vi "InsertData.vi"(4 "Mag B":dbl, 6 "Temp T":dbl, 7 "Time Stamp":timestamp, 8 "error in (no error)":errorcluster, 10 "VNACluster In":T1={"Value"=0.0, "GUI Data Cluster"={"S11"=FALSE, "S21"=FALSE, "S12"=FALSE, "S22"=FALSE, "S11Meas"=enum."Log-magnitude (dB)", "S21Meas"=enum."Log-magnitude (dB)", "S12Meas"=enum."Log-magnitude (dB)", "S22Meas"=enum."Log-magnitude (dB)"}, "Timing"={"Last Operation"=0.0, "Stop @ T"=FALSE, "Delta T Log"=FALSE, "End T"=0.0, "Delta T"=0.0, "Last Temp"=0.0}, "Measurements"=[], "Hardware"={"VNA TCP Con"=refnum, "VNA TCP Port"=5025, "Global T VAR"="", "Global B VAR"=""}, "Operation"={"Operation Mode"=enum."Logging", "Log Folder"=path "", "Measure Mode"=enum."Deltat"}}) -> (0 "error out":errorcluster, 2 "VNACluster Out":T1={"Value"=0.0, "GUI Data Cluster"={"S11"=FALSE, "S21"=FALSE, "S12"=FALSE, "S22"=FALSE, "S11Meas"=enum."Log-magnitude (dB)", "S21Meas"=enum."Log-magnitude (dB)", "S12Meas"=enum."Log-magnitude (dB)", "S22Meas"=enum."Log-magnitude (dB)"}, "Timing"={"Last Operation"=0.0, "Stop @ T"=FALSE, "Delta T Log"=FALSE, "End T"=0.0, "Delta T"=0.0, "Last Temp"=0.0}, "Measurements"=[], "Hardware"={"VNA TCP Con"=refnum, "VNA TCP Port"=5025, "Global T VAR"="", "Global B VAR"=""}, "Operation"={"Operation Mode"=enum."Logging", "Log Folder"=path "", "Measure Mode"=enum."Deltat"}})   [LabVIEW 2021]
uses:
  Sources/Data_Cluster.ctl
  Sources/Measurement_Cluster.ctl
  Sources/Mode_Enum.ctl
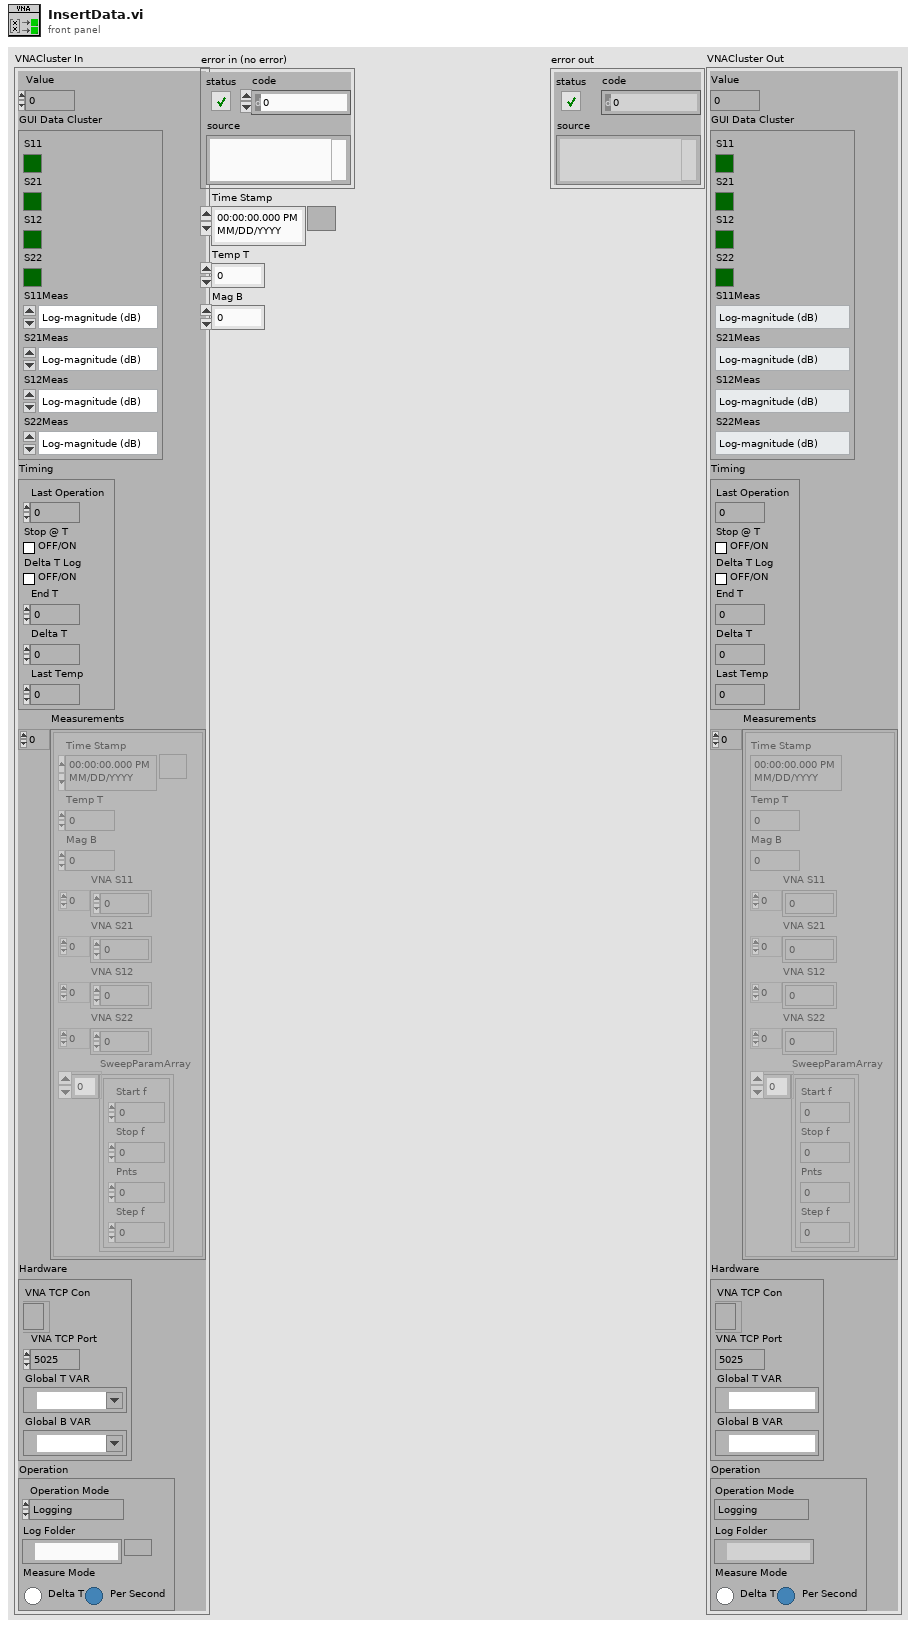
[diagram p1: front panel]
types:
  T1 = typedef "Data_Cluster.ctl" = cluster{"Value":dbl, "GUI Data Cluster":cluster{"S11":bool, "S21":bool, "S12":bool, "S22":bool, "S11Meas":enum16{"Log-magnitude (dB)", "Linear magnitude", "Phase (deg)", "Time Domain", "Real", "Imaginary", "Group Delay", "Polarlinear"}, "S21Meas":enum16{"Log-magnitude (dB)", "Linear magnitude", "Phase (deg)", "Time Domain", "Real", "Imaginary", "Group Delay", "Polarlinear"}, "S12Meas":enum16{"Log-magnitude (dB)", "Linear magnitude", "Phase (deg)", "Time Domain", "Real", "Imaginary", "Group Delay", "Polarlinear"}, "S22Meas":enum16{"Log-magnitude (dB)", "Linear magnitude", "Phase (deg)", "Time Domain", "Real", "Imaginary", "Group Delay", "Polarlinear"}}, "Timing":cluster{"Last Operation":dbl, "Stop @ T":bool, "Delta T Log":bool, "End T":dbl, "Delta T":dbl, "Last Temp":dbl}, "Measurements":T2[], "Hardware":cluster{"VNA TCP Con":refnum<k5>, "VNA TCP Port":i32, "Global T VAR":refnum<k21>, "Global B VAR":refnum<k21>}, "Operation":cluster{"Operation Mode":T3, "Log Folder":path, "Measure Mode":enum32{"DeltaT", "Deltat"}}}
  T2 = typedef "Measurement_Cluster.ctl" = cluster{"Time Stamp":timestamp, "Temp T":dbl, "Mag B":dbl, "VNA S11":dbl[], "VNA S21":dbl[], "VNA S12":dbl[], "VNA S22":dbl[], "SweepParamArray":cluster{"Start f":dbl, "Stop f":dbl, "Pnts":i32, "Step f":dbl}[]}
  T3 = typedef "Mode_Enum.ctl" = enum16{"Logging", "Idle-Off", "Idle"}
  T4 = cluster{"S11":bool, "S21":bool, "S12":bool, "S22":bool, "S11Meas":enum16{"Log-magnitude (dB)", "Linear magnitude", "Phase (deg)", "Time Domain", "Real", "Imaginary", "Group Delay", "Polarlinear"}, "S21Meas":enum16{"Log-magnitude (dB)", "Linear magnitude", "Phase (deg)", "Time Domain", "Real", "Imaginary", "Group Delay", "Polarlinear"}, "S12Meas":enum16{"Log-magnitude (dB)", "Linear magnitude", "Phase (deg)", "Time Domain", "Real", "Imaginary", "Group Delay", "Polarlinear"}, "S22Meas":enum16{"Log-magnitude (dB)", "Linear magnitude", "Phase (deg)", "Time Domain", "Real", "Imaginary", "Group Delay", "Polarlinear"}}
  T5 = enum16{"Log-magnitude (dB)", "Linear magnitude", "Phase (deg)", "Time Domain", "Real", "Imaginary", "Group Delay", "Polarlinear"}
  T6 = enum16{"Log-magnitude (dB)", "Linear magnitude", "Phase (deg)", "Time Domain", "Real", "Imaginary", "Group Delay", "Polarlinear"}[]
  T7 = cluster{"Start f":dbl, "Stop f":dbl, "Pnts":i32, "Step f":dbl}
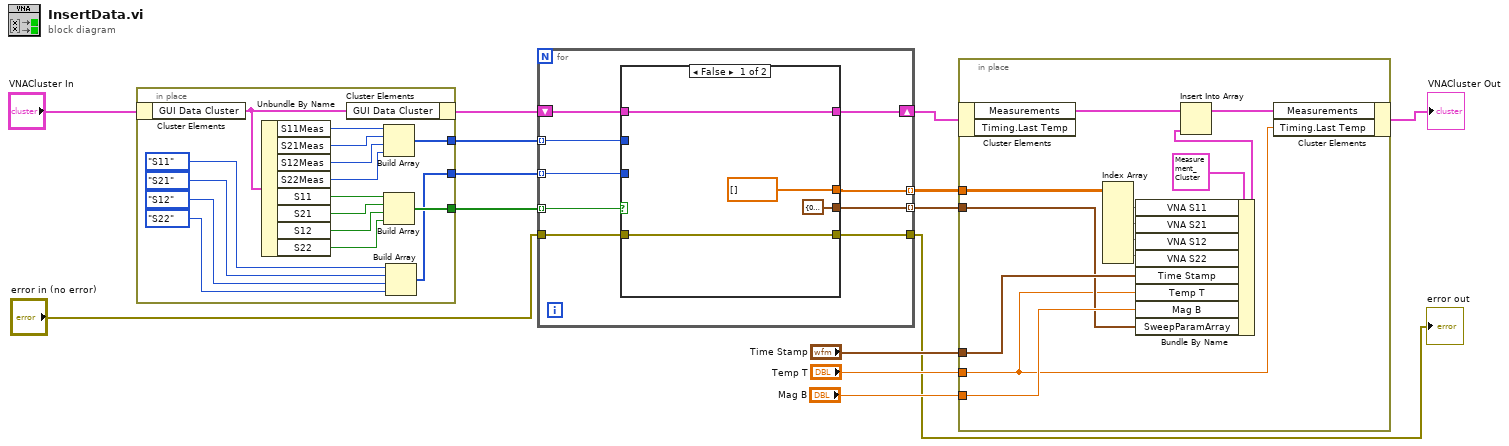
[diagram p0: block diagram]
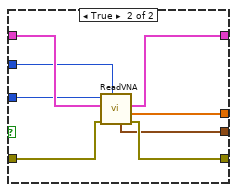
[diagram p2: hidden frame]
diagram:
  n1 = in-place {
    in-place-border: [w21] -> w13
    in-place-border: [w20] -> w12
    in-place-border: [w15] -> w9
    n2 = in-place-cluster #1("VNACluster In") -> ("GUI Data Cluster"=w30:T4)
    n3 = Unbundle By Name(w30) -> ("S11Meas"=w29:T5, "S21Meas"=w28:T5, "S12Meas"=w27:T5, "S22Meas"=w26:T5, "S11"=w25:bool, "S21"=w24:bool, "S12"=w23:bool, "S22"=w22:bool)
    n4 = in-place-cluster #1("GUI Data Cluster"=w30) -> (w11:T1)
    n5 = Build Array(w29, w28, w27, w26) -> (w21:T6)
    n6 = Build Array(w25, w24, w23, w22) -> (w20:bool[])
    n7 = Build Array(enum16{"S11", "S21", "S12", "S22"}."S11" ("Param"), enum16{"S11", "S21", "S12", "S22"}."S21" ("Param"), enum16{"S11", "S21", "S12", "S22"}."S12" ("Param"), enum16{"S11", "S21", "S12", "S22"}."S22" ("Param")) -> (w15:enum16{"S11", "S21", "S12", "S22"}[])
  }
  n8 = for {
    tunnel: w13 -> [w35] mode=indexing
    tunnel: w12 -> [w36] mode=indexing
    tunnel: "error in (no error)" -> [w38]
    tunnel: w9 -> [w37] mode=indexing
    shift-right: [w34] -> w8
    shift-left: w11 -> [w39]
    tunnel: [w33] -> w2
    tunnel: [w32] -> w7 mode=indexing
    tunnel: [w31] -> w1 mode=indexing
    n9 = case shown="False" w36 {
      tunnel: w39 -> [w43 w51]
      tunnel: w38 -> [w42 w50]
      tunnel: w37 -> [_ w49]
      tunnel: w35 -> [_ w48]
      tunnel: [w43 w47] -> w34
      tunnel: [dbl[] [] w46] -> w32
      tunnel: [w42 w45] -> w33
      tunnel: [T7 {"Start f"=0.0, "Stop f"=0.0, "Pnts"=0, "Step f"=0.0} ("SweepParam") w44] -> w31
      frame False {
      }
      frame True {
        n10 = call "ReadVNA.vi"("Data Type"=w48, "error in (no error)"=w50, "VNACluster In"=w51, "Param"=w49) -> ("error out"=w45:errorcluster, "Array"=w46:dbl[], "VNACluster Out"=w47:T1, "SweepParam"=w44:T7)  [unwired: 4 in]
      }
    }
  }
  "error out" <- w2
  n11 = in-place {
    in-place-border: w7 -> [w60]
    in-place-border: "Time Stamp" -> [w55]
    in-place-border: "Temp T" -> [w52]
    in-place-border: "Mag B" -> [w54]
    in-place-border: w1 -> [w53]
    n12 = in-place-cluster #2(w8) -> ("Measurements"=w64:T2[])  [unwired: 1 out]
    n13 = Index Array(array=w60) -> (element #1=w59:dbl[], element #2=w58:dbl[], element #3=w57:dbl[], element #4=w56:dbl[])  [unwired: 8 in]
    n14 = Bundle By Name(cluster=T2 {"Time Stamp"=timestamp(0 s since 1904-01-01), "Temp T"=0.0, "Mag B"=0.0, "VNA S11"=[], "VNA S21"=[], "VNA S12"=[], "VNA S22"=[], "SweepParamArray"=[]} ("new element/subarray"), "VNA S11"=w59, "VNA S21"=w58, "VNA S12"=w57, "VNA S22"=w56, "Time Stamp"=w55, "Temp T"=w52, "Mag B"=w54, "SweepParamArray"=w53) -> (w61:T2)
    n15 = Insert Into Array(array=w64, new element=w61) -> (w63:T2[])  [unwired: 1 in]
    n16 = in-place-cluster #2("Measurements"=w63, "Timing.Last Temp"=w52) -> (→"VNACluster Out":T1)
  }
